vi "OEE_SCREEN_2_calculate_cycle_time_exceeded.vi"(2 "cycle_time_actual":string, 3 "cycle_time_target":string) -> (0 "target_actual_seconds_over":i32[](array[numeric]))   [LabVIEW 2019]
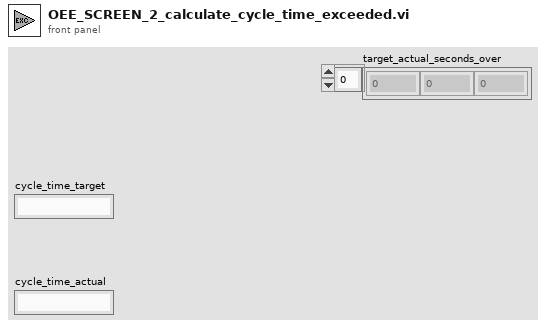
[diagram p1: front panel]
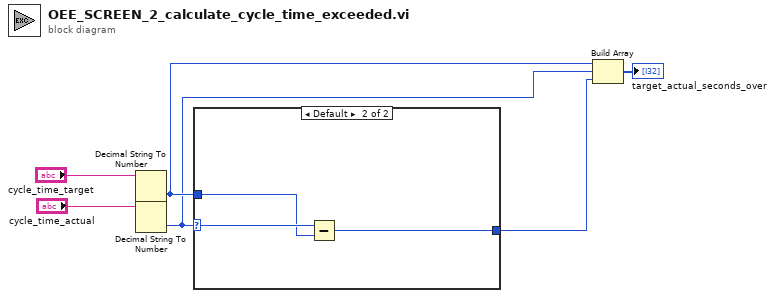
[diagram p0: block diagram]
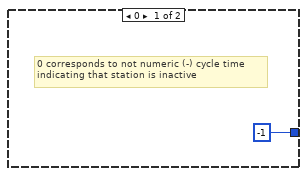
[diagram p2: hidden frame]
diagram:
  n1 = Decimal String To Number(string="cycle_time_target") -> (number=w4:i32)  [unwired: 2 in, 1 out]
  n2 = Decimal String To Number(string="cycle_time_actual") -> (number=w3:i32)  [unwired: 2 in, 1 out]
  n3 = case shown="Default" w3 {
    selector: w3 -> [_ w10]
    tunnel: [-1 ("seconds_over_cycle_time") w8] -> w2
    tunnel: w4 -> [_ w9]
    frame 0 {
      # "0 corresponds to not numeric (-) cycle time\nindicating that station is inactive"
    }
    frame Default {
      n4 = Subtract(x=w10, y=w9) -> (x-y=w8:i32)
    }
  }
  n5 = Build Array(w4, w3, w2) -> (→"target_actual_seconds_over":i32[])
